vi "Read log file.vi"() -> ()   [LabVIEW 2013]
panel:
  out "XY Graph":cluster{timestamp, u8, dbl}[](graph)
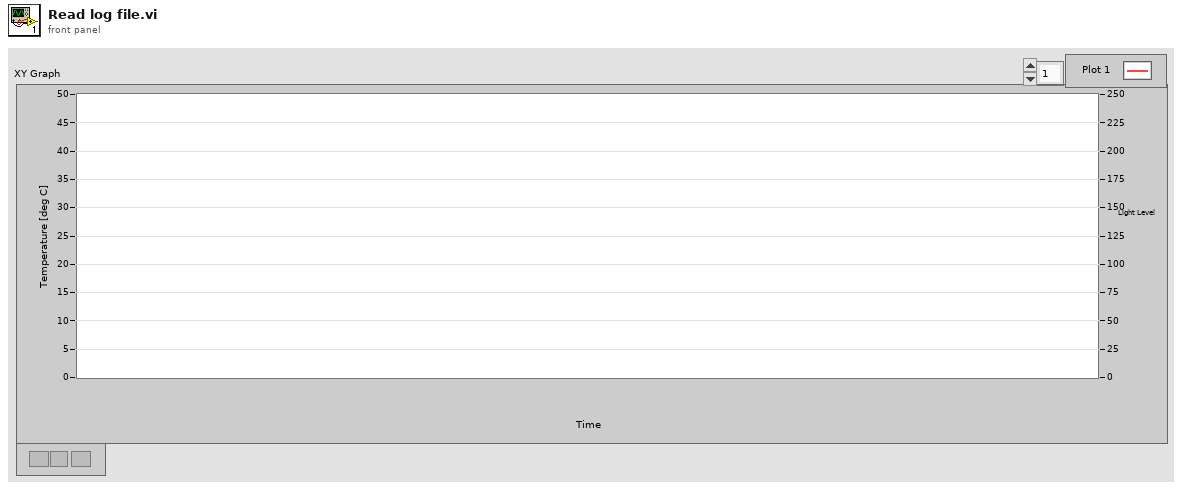
[diagram p1: front panel]
types:
  T1 = enum16{"open", "replace", "create", "open or create", "replace or create", "replace or create with confirmation"}
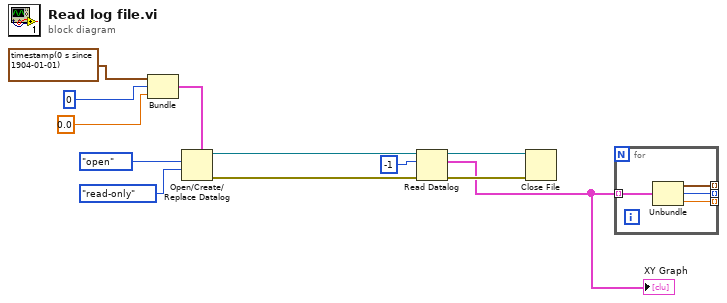
[diagram p0: block diagram]
diagram:
  n1 = Bundle(timestamp(0 s since 1904-01-01), u8 0, 0.0) -> (w7:cluster{timestamp, u8, dbl})  [unwired: 1 in]
  n2 = Open/Create/Replace Datalog(5:w7, 9:enum16{"read/write", "read-only", "write-only"}."read-only" ("access (0:read/write)"), 10:T1."open" ("operation (0:open)")) -> (0:w4:errorcluster, 3:w5:refnum<k1>)  [unwired: 3 in, 1 out]
  n3 = Read Datalog(4:w4, 6:-1 ("count (1)"), 7:w5) -> (0:w2:errorcluster, 2:w1:cluster{timestamp, u8, dbl}[], 3:w3:refnum<k1>)
  "XY Graph" <- w1
  n4 = Close File(refnum=w3, error in=w2) -> ()  [unwired: 2 out]
  n5 = for {
    tunnel: w1 -> [w16] mode=indexing
    tunnel: [w15] -> _ mode=indexing
    tunnel: [w14] -> _ mode=indexing
    tunnel: [w13] -> _ mode=indexing
    n6 = Unbundle(w16) -> (w15:timestamp, w14:u8, w13:dbl)
  }
